vi "health_parameters.vi"(8 "error in\n(no error)":errorcluster, 10 "parameters":string[][](array[string]), 11 "hDin":T1={"nSignals"=0, "logname"="", "time"=timestamp(0 s since 1904-01-01), "dir"=path "", "adamSerial"={"port"="COM1", "timeout"=1000, "baud"=9600, "dataBits"=8, "stopBits"=10, "flowControl"=0, "parity"=0, "termChar"=FALSE, "checkSum"=FALSE}, "fiberSerial"={"port1"="COM1", "port2"="COM1", "timeout"=1000, "baud"=9600, "dataBits"=8, "stopBits"=10, "flowControl"=0, "parity"=0, "termChar"=FALSE, "checkSum"=FALSE, "fiber1On"=FALSE, "fiber2On"=FALSE}, "signal"={"src"=[], "id"=[], "ch"=[], "descrip"=[], "units"=[], "scale"=[], "hi"=[], "lo"=[], "rec"=[], "fault"=[], "val"=[]}, "teSerial"={"port"="COM1", "timeout"=1000, "baud"=9600, "dataBits"=8, "stopBits"=10, "flowControl"=0, "parity"=0, "termChar"=FALSE, "checkSum"=FALSE, "checkSumVal"=""}, "lograte"=0, "calSwitch"=FALSE, "logoffset"=0.0} {"teSerial"."stopBits" items=["1.0"=10, "1.5"=15, "2.0"=20]; "teSerial"."parity" items=["None", "Odd", "Even", "Mark", "Space"]; "teSerial"."flowControl" items=["None"=0, "XON/XOFF"=1, "RTS/CTS"=2, "DTR/DSR"=4]; "fiberSerial"."stopBits" items=["1.0"=10, "1.5"=15, "2.0"=20]; "fiberSerial"."parity" items=["None", "Odd", "Even", "Mark", "Space"]; "fiberSerial"."flowControl" items=["None"=0, "XON/XOFF"=1, "RTS/CTS"=2, "DTR/DSR"=4]; "adamSerial"."stopBits" items=["1.0"=10, "1.5"=15, "2.0"=20]; "adamSerial"."parity" items=["None", "Odd", "Even", "Mark", "Space"]; "adamSerial"."flowControl" items=["None"=0, "XON/XOFF"=1, "RTS/CTS"=2, "DTR/DSR"=4]}) -> (0 "error out":errorcluster, 3 "hDout":T1={"nSignals"=0, "logname"="", "time"=timestamp(0 s since 1904-01-01), "dir"=path "", "adamSerial"={"port"="COM1", "timeout"=1000, "baud"=9600, "dataBits"=8, "stopBits"=10, "flowControl"=0, "parity"=0, "termChar"=FALSE, "checkSum"=FALSE}, "fiberSerial"={"port1"="COM1", "port2"="COM1", "timeout"=1000, "baud"=9600, "dataBits"=8, "stopBits"=10, "flowControl"=0, "parity"=0, "termChar"=FALSE, "checkSum"=FALSE, "fiber1On"=FALSE, "fiber2On"=FALSE}, "signal"={"src"=[], "id"=[], "ch"=[], "descrip"=[], "units"=[], "scale"=[], "hi"=[], "lo"=[], "rec"=[], "fault"=[], "val"=[]}, "teSerial"={"port"="COM1", "timeout"=1000, "baud"=9600, "dataBits"=8, "stopBits"=10, "flowControl"=0, "parity"=0, "termChar"=FALSE, "checkSum"=FALSE, "checkSumVal"=""}, "lograte"=0, "calSwitch"=FALSE, "logoffset"=0.0} {"teSerial"."stopBits" items=["1.0"=10, "1.5"=15, "2.0"=20]; "teSerial"."parity" items=["None", "Odd", "Even", "Mark", "Space"]; "teSerial"."flowControl" items=["None"=0, "XON/XOFF"=1, "RTS/CTS"=2, "DTR/DSR"=4]; "fiberSerial"."stopBits" items=["1.0"=10, "1.5"=15, "2.0"=20]; "fiberSerial"."parity" items=["None", "Odd", "Even", "Mark", "Space"]; "fiberSerial"."flowControl" items=["None"=0, "XON/XOFF"=1, "RTS/CTS"=2, "DTR/DSR"=4]; "adamSerial"."stopBits" items=["1.0"=10, "1.5"=15, "2.0"=20]; "adamSerial"."parity" items=["None", "Odd", "Even", "Mark", "Space"]; "adamSerial"."flowControl" items=["None"=0, "XON/XOFF"=1, "RTS/CTS"=2, "DTR/DSR"=4]})   [LabVIEW 2018]
uses:
  health_Loop_Clust.ctl
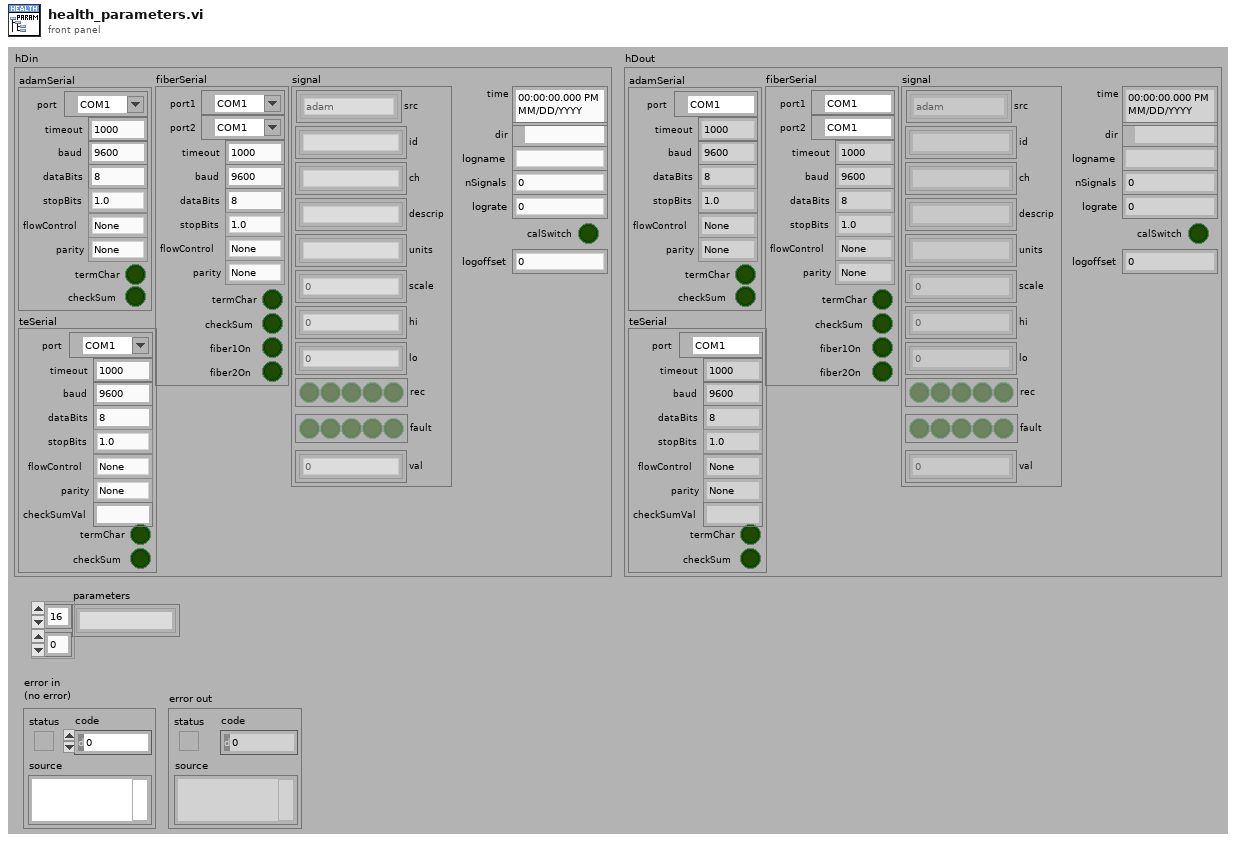
[diagram p1: front panel]
types:
  T1 = typedef "health_Loop_Clust.ctl" = cluster{"nSignals":i32, "logname":string, "time":timestamp, "dir":path, "adamSerial":cluster{"port":refnum<visa-resource-name>, "timeout":u32, "baud":u32, "dataBits":u16, "stopBits":u16, "flowControl":u16, "parity":u16, "termChar":bool, "checkSum":bool}, "fiberSerial":cluster{"port1":refnum<visa-resource-name>, "port2":refnum<visa-resource-name>, "timeout":u32, "baud":u32, "dataBits":u16, "stopBits":u16, "flowControl":u16, "parity":u16, "termChar":bool, "checkSum":bool, "fiber1On":bool, "fiber2On":bool}, "signal":cluster{"src":enum16{"adam", "fiber", "te"}[], "id":string[], "ch":string[], "descrip":string[], "units":string[], "scale":dbl[], "hi":dbl[], "lo":dbl[], "rec":bool[], "fault":bool[], "val":dbl[]}, "teSerial":cluster{"port":refnum<visa-resource-name>, "timeout":u32, "baud":u32, "dataBits":u16, "stopBits":u16, "flowControl":u16, "parity":u16, "termChar":bool, "checkSum":bool, "checkSumVal":string}, "lograte":u32, "calSwitch":bool, "logoffset":dbl}
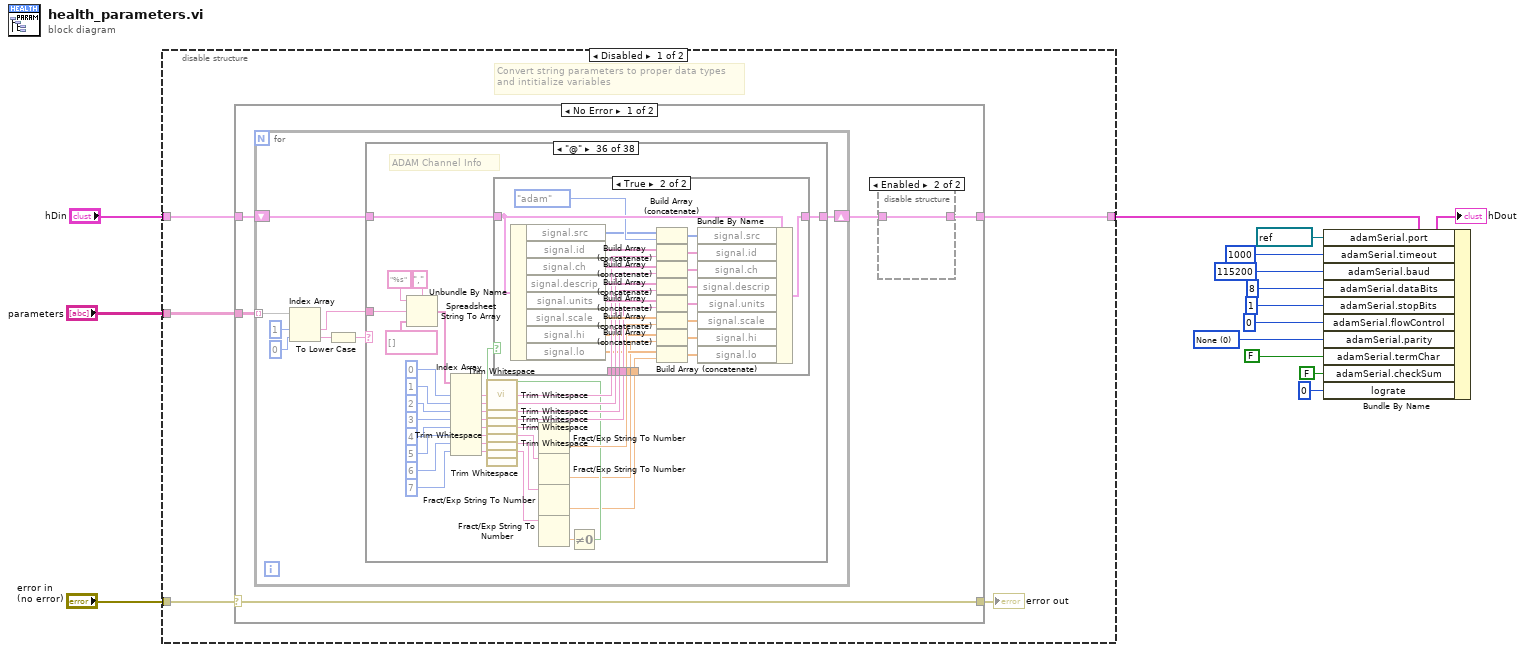
[diagram p0: block diagram]
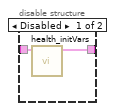
[diagram p2: hidden frame]
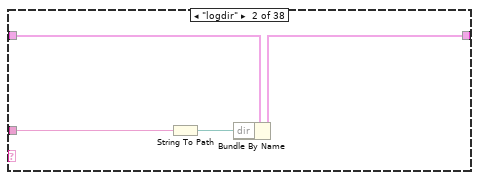
[diagram p4: hidden frame]
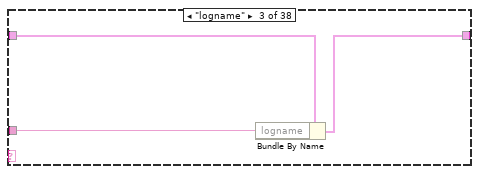
[diagram p5: hidden frame]
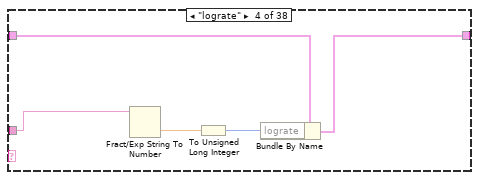
[diagram p6: hidden frame]
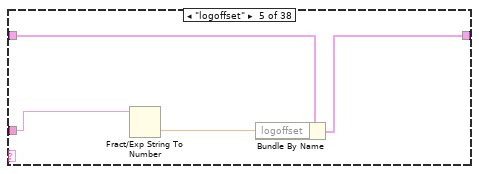
[diagram p7: hidden frame]
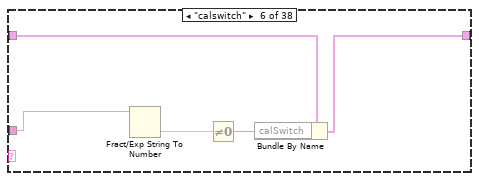
[diagram p8: hidden frame]
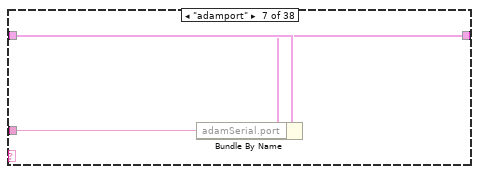
[diagram p9: hidden frame]
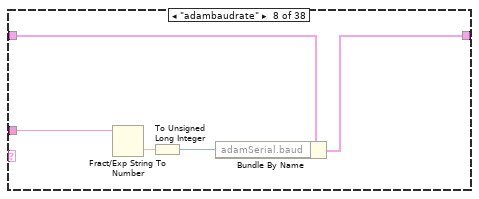
[diagram p10: hidden frame]
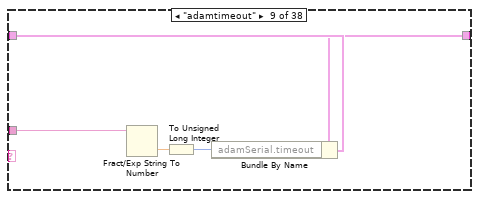
[diagram p11: hidden frame]
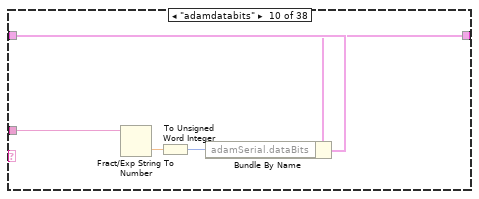
[diagram p12: hidden frame]
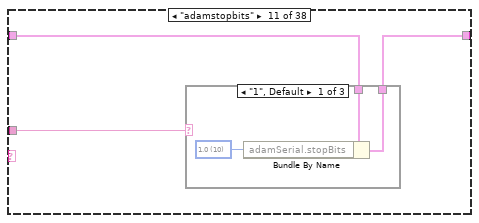
[diagram p13: hidden frame]
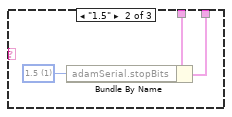
[diagram p14: hidden frame]
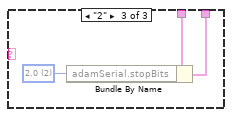
[diagram p15: hidden frame]
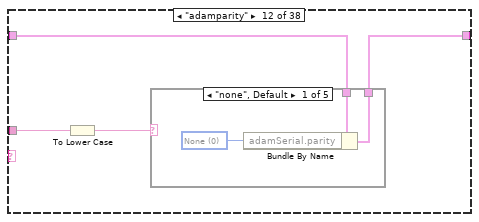
[diagram p16: hidden frame]
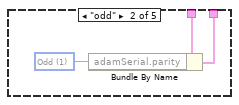
[diagram p17: hidden frame]
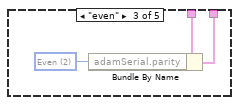
[diagram p18: hidden frame]
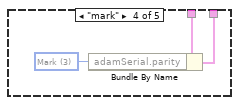
[diagram p19: hidden frame]
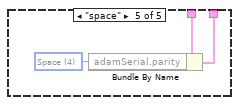
[diagram p20: hidden frame]
diagram:
  w1 = u16 0 items=["None", "Odd", "Even", "Mark", "Space"] ("parity")
  n1 = disable-structure shown="Disabled" {
    disable-tunnel: "error in\n(no error)" -> [w20 _]
    disable-tunnel: "parameters" -> [w18 _]
    disable-tunnel: "hDin" -> [w17 w487]
    disable-tunnel: [w16 w487] -> w12
    frame Disabled {
      # "Convert string parameters to proper data types\nand intitialize variables"
      n2 = case shown="No Error" w20 {
        selector: w20 -> [w25 w486]
        tunnel: [w25 w486] -> w19
        tunnel: [w21 w485] -> w16
        tunnel: w17 -> [w23 w485]
        tunnel: w18 -> [w24 _]
        frame No Error {
          n3 = for {
            shift-right: [w29] -> w22
            shift-left: w23 -> [w30]
            tunnel: w24 -> [w36] mode=indexing
            n4 = Index Array(array=w36, index #1=1 ("index"), index #2=0 ("index")) -> (element #1=w33:string, element #2=w32:string)
            n5 = To Lower Case(string=w32) -> (all lower case string=w31:string)
            n6 = case shown="\"@\"" w31 {
              tunnel: [w37 w40 w43 w48 w52 w57 w60 w65 w68 w73 w78 w91 w110 w128 w134 w137 w140 w145 w148 w153 w158 w171 w190 w208 w214 w217 w222 w225 w230 w235 w248 w267 w285 w291 w294 w319 w382 w445] -> w29
              tunnel: w33 -> [_ w39 w42 w47 w51 w56 w59 w66 w67 w75 w77 w90 w109 w127 w133 w136 w139 w146 w147 w155 w157 w170 w189 w207 w213 w216 w223 w224 w232 w234 w247 w266 w284 w290 w293 w328 w391 w454]
              tunnel: w30 -> [w37 w41 w44 w49 w53 w58 w61 w63 w69 w74 w79 w92 w111 w129 w135 w138 w141 w143 w149 w154 w159 w172 w191 w209 w215 w218 w220 w226 w231 w236 w249 w268 w286 w292 w295 w326 w389 w452]
              frame Default {
                # "Parameter Not Recognized"
              }
              frame "logdir" {
                n7 = String To Path(string=w39) -> (path=w38:path)
                n8 = Bundle By Name(cluster=w41, "dir"=w38) -> (w40:T1)
              }
              frame "logname" {
                n9 = Bundle By Name(cluster=w44, "logname"=w42) -> (w43:T1)
              }
              frame "lograte" {
                n10 = Fract/Exp String To Number(string=w47) -> (number=w45:dbl)  [unwired: 3 in, 1 out]
                n11 = To Unsigned Long Integer(number=w45) -> (unsigned 32bit integer=w46:u32)
                n12 = Bundle By Name(cluster=w49, "lograte"=w46) -> (w48:T1)
              }
              frame "logoffset" {
                n13 = Fract/Exp String To Number(string=w51) -> (number=w50:dbl)  [unwired: 3 in, 1 out]
                n14 = Bundle By Name(cluster=w53, "logoffset"=w50) -> (w52:T1)
              }
              frame "calswitch" {
                n15 = Fract/Exp String To Number(string=w56) -> (number=w54:dbl)  [unwired: 3 in, 1 out]
                n16 = Not Equal To 0?(x=w54) -> (x != 0?=w55:bool)
                n17 = Bundle By Name(cluster=w58, "calSwitch"=w55) -> (w57:T1)
              }
              frame "adamport" {
                n18 = Bundle By Name(cluster=w61, "adamSerial.port"=w59) -> (w60:T1)
              }
              frame "adambaudrate" {
                n19 = Fract/Exp String To Number(string=w66) -> (number=w64:dbl)  [unwired: 3 in, 1 out]
                n20 = To Unsigned Long Integer(number=w64) -> (unsigned 32bit integer=w62:u32)
                n21 = Bundle By Name(cluster=w63, "adamSerial.baud"=w62) -> (w65:T1)
              }
              frame "adamtimeout" {
                n22 = Fract/Exp String To Number(string=w67) -> (number=w70:dbl)  [unwired: 3 in, 1 out]
                n23 = To Unsigned Long Integer(number=w70) -> (unsigned 32bit integer=w71:u32)
                n24 = Bundle By Name(cluster=w69, "adamSerial.timeout"=w71) -> (w68:T1)
              }
              frame "adamdatabits" {
                n25 = Fract/Exp String To Number(string=w75) -> (number=w76:dbl)  [unwired: 3 in, 1 out]
                n26 = To Unsigned Word Integer(number=w76) -> (unsigned 16bit integer=w72:u16)
                n27 = Bundle By Name(cluster=w74, "adamSerial.dataBits"=w72) -> (w73:T1)
              }
              frame "adamstopbits" {
                n28 = case shown="\"1\", Default" w77 {
                  tunnel: w79 -> [w82 w85 w88]
                  tunnel: [w81 w84 w87] -> w78
                  frame "1", Default {
                    w80 = u16 10 items=["1.0"=10, "1.5"=15, "2.0"=20] ("stopBits")
                    n29 = Bundle By Name(cluster=w82, "adamSerial.stopBits"=w80) -> (w81:T1)
                  }
                  frame "1.5" {
                    w83 = u16 1 items=["1.0", "1.5", "2.0", "Other"] ("stopBits")
                    n30 = Bundle By Name(cluster=w85, "adamSerial.stopBits"=w83) -> (w84:T1)
                  }
                  frame "2" {
                    w86 = u16 2 items=["1.0", "1.5", "2.0", "Other"] ("stopBits")
                    n31 = Bundle By Name(cluster=w88, "adamSerial.stopBits"=w86) -> (w87:T1)
                  }
                }
              }
              frame "adamparity" {
                n32 = To Lower Case(string=w90) -> (all lower case string=w89:string)
                n33 = case shown="\"none\", Default" w89 {
                  tunnel: w92 -> [w95 w98 w101 w104 w107]
                  tunnel: [w94 w97 w100 w103 w106] -> w91
                  frame "none", Default {
                    w93 = u16 0 items=["None", "Odd", "Even", "Mark", "Space"] ("parity")
                    n34 = Bundle By Name(cluster=w95, "adamSerial.parity"=w93) -> (w94:T1)
                  }
                  frame "odd" {
                    w96 = u16 1 items=["None", "Odd", "Even", "Mark", "Space"] ("parity")
                    n35 = Bundle By Name(cluster=w98, "adamSerial.parity"=w96) -> (w97:T1)
                  }
                  frame "even" {
                    w99 = u16 2 items=["None", "Odd", "Even", "Mark", "Space"] ("parity")
                    n36 = Bundle By Name(cluster=w101, "adamSerial.parity"=w99) -> (w100:T1)
                  }
                  frame "mark" {
                    w102 = u16 3 items=["None", "Odd", "Even", "Mark", "Space"] ("parity")
                    n37 = Bundle By Name(cluster=w104, "adamSerial.parity"=w102) -> (w103:T1)
                  }
                  frame "space" {
                    w105 = u16 4 items=["None", "Odd", "Even", "Mark", "Space"] ("parity")
                    n38 = Bundle By Name(cluster=w107, "adamSerial.parity"=w105) -> (w106:T1)
                  }
                }
              }
              frame "adamflowcontrol" {
                n39 = To Lower Case(string=w109) -> (all lower case string=w108:string)
                n40 = case shown="\"none\", Default" w108 {
                  tunnel: w111 -> [w114 w117 w120 w123]
                  tunnel: [w113 w116 w119 w122] -> w110
                  frame "none", Default {
                    w112 = u16 0 items=["None"=0, "XON/XOFF"=1, "RTS/CTS"=2, "DTR/DSR"=4] ("flowControl")
                    n41 = Bundle By Name(cluster=w114, "adamSerial.flowControl"=w112) -> (w113:T1)
                  }
                  frame "xon/xoff" {
                    w115 = u16 1 items=["None"=0, "XON/XOFF"=1, "RTS/CTS"=2, "DTR/DSR"=4] ("flowControl")
                    n42 = Bundle By Name(cluster=w117, "adamSerial.flowControl"=w115) -> (w116:T1)
                  }
                  frame "rts/cts" {
                    w118 = u16 2 items=["None"=0, "XON/XOFF"=1, "RTS/CTS"=2, "DTR/DSR"=4] ("flowControl")
                    n43 = Bundle By Name(cluster=w120, "adamSerial.flowControl"=w118) -> (w119:T1)
                  }
                  frame "dtr/dsr" {
                    w121 = u16 4 items=["None"=0, "XON/XOFF"=1, "RTS/CTS"=2, "DTR/DSR"=4] ("flowControl")
                    n44 = Bundle By Name(cluster=w123, "adamSerial.flowControl"=w121) -> (w122:T1)
                  }
                }
              }
              frame "adamtermchar" {
                n45 = Fract/Exp String To Number(string=w127) -> (number=w126:dbl)  [unwired: 3 in, 1 out]
                n46 = Equal?(x=w126, y=1.0) -> (x = y?=w124:bool)
                n47 = Bundle By Name(cluster=w129, "adamSerial.termChar"=w124) -> (w128:T1)
              }
              frame "adamchecksum" {
                n48 = Fract/Exp String To Number(string=w133) -> (number=w132:dbl)  [unwired: 3 in, 1 out]
                n49 = Equal?(x=w132, y=1.0) -> (x = y?=w130:bool)
                n50 = Bundle By Name(cluster=w135, "adamSerial.checkSum"=w130) -> (w134:T1)
              }
              frame "fiberport1" {
                n51 = Bundle By Name(cluster=w138, "fiberSerial.port1"=w136) -> (w137:T1)
              }
              frame "fiberport2" {
                n52 = Bundle By Name(cluster=w141, "fiberSerial.port2"=w139) -> (w140:T1)
              }
              frame "fiberbaudrate" {
                n53 = Fract/Exp String To Number(string=w146) -> (number=w144:dbl)  [unwired: 3 in, 1 out]
                n54 = To Unsigned Long Integer(number=w144) -> (unsigned 32bit integer=w142:u32)
                n55 = Bundle By Name(cluster=w143, "fiberSerial.baud"=w142) -> (w145:T1)
              }
              frame "fibertimeout" {
                n56 = Fract/Exp String To Number(string=w147) -> (number=w150:dbl)  [unwired: 3 in, 1 out]
                n57 = To Unsigned Long Integer(number=w150) -> (unsigned 32bit integer=w151:u32)
                n58 = Bundle By Name(cluster=w149, "fiberSerial.timeout"=w151) -> (w148:T1)
              }
              frame "fiberdatabits" {
                n59 = Fract/Exp String To Number(string=w155) -> (number=w156:dbl)  [unwired: 3 in, 1 out]
                n60 = To Unsigned Word Integer(number=w156) -> (unsigned 16bit integer=w152:u16)
                n61 = Bundle By Name(cluster=w154, "fiberSerial.dataBits"=w152) -> (w153:T1)
              }
              frame "fiberstopbits" {
                n62 = case shown="\"1\", Default" w157 {
                  tunnel: w159 -> [w162 w165 w168]
                  tunnel: [w161 w164 w167] -> w158
                  frame "1", Default {
                    w160 = u16 10 items=["1.0"=10, "1.5"=15, "2.0"=20] ("stopBits")
                    n63 = Bundle By Name(cluster=w162, "fiberSerial.stopBits"=w160) -> (w161:T1)
                  }
                  frame "1.5" {
                    w163 = u16 1 items=["1.0", "1.5", "2.0", "Other"] ("stopBits")
                    n64 = Bundle By Name(cluster=w165, "fiberSerial.stopBits"=w163) -> (w164:T1)
                  }
                  frame "2" {
                    w166 = u16 2 items=["1.0", "1.5", "2.0", "Other"] ("stopBits")
                    n65 = Bundle By Name(cluster=w168, "fiberSerial.stopBits"=w166) -> (w167:T1)
                  }
                }
              }
              frame "fiberparity" {
                n66 = To Lower Case(string=w170) -> (all lower case string=w169:string)
                n67 = case shown="\"none\", Default" w169 {
                  tunnel: w172 -> [w175 w178 w181 w184 w187]
                  tunnel: [w174 w177 w180 w183 w186] -> w171
                  frame "none", Default {
                    w173 = u16 0 items=["None", "Odd", "Even", "Mark", "Space"] ("parity")
                    n68 = Bundle By Name(cluster=w175, "fiberSerial.parity"=w173) -> (w174:T1)
                  }
                  frame "odd" {
                    w176 = u16 1 items=["None", "Odd", "Even", "Mark", "Space"] ("parity")
                    n69 = Bundle By Name(cluster=w178, "fiberSerial.parity"=w176) -> (w177:T1)
                  }
                  frame "even" {
                    w179 = u16 2 items=["None", "Odd", "Even", "Mark", "Space"] ("parity")
                    n70 = Bundle By Name(cluster=w181, "fiberSerial.parity"=w179) -> (w180:T1)
                  }
                  frame "mark" {
                    w182 = u16 3 items=["None", "Odd", "Even", "Mark", "Space"] ("parity")
                    n71 = Bundle By Name(cluster=w184, "fiberSerial.parity"=w182) -> (w183:T1)
                  }
                  frame "space" {
                    w185 = u16 4 items=["None", "Odd", "Even", "Mark", "Space"] ("parity")
                    n72 = Bundle By Name(cluster=w187, "fiberSerial.parity"=w185) -> (w186:T1)
                  }
                }
              }
              frame "fiberflowcontrol" {
                n73 = To Lower Case(string=w189) -> (all lower case string=w188:string)
                n74 = case shown="\"none\", Default" w188 {
                  tunnel: w191 -> [w194 w197 w200 w203]
                  tunnel: [w193 w196 w199 w202] -> w190
                  frame "none", Default {
                    w192 = u16 0 items=["None"=0, "XON/XOFF"=1, "RTS/CTS"=2, "DTR/DSR"=4] ("flowControl")
                    n75 = Bundle By Name(cluster=w194, "fiberSerial.flowControl"=w192) -> (w193:T1)
                  }
                  frame "xon/xoff" {
                    w195 = u16 1 items=["None"=0, "XON/XOFF"=1, "RTS/CTS"=2, "DTR/DSR"=4] ("flowControl")
                    n76 = Bundle By Name(cluster=w197, "fiberSerial.flowControl"=w195) -> (w196:T1)
                  }
                  frame "rts/cts" {
                    w198 = u16 2 items=["None"=0, "XON/XOFF"=1, "RTS/CTS"=2, "DTR/DSR"=4] ("flowControl")
                    n77 = Bundle By Name(cluster=w200, "fiberSerial.flowControl"=w198) -> (w199:T1)
                  }
                  frame "dtr/dsr" {
                    w201 = u16 4 items=["None"=0, "XON/XOFF"=1, "RTS/CTS"=2, "DTR/DSR"=4] ("flowControl")
                    n78 = Bundle By Name(cluster=w203, "fiberSerial.flowControl"=w201) -> (w202:T1)
                  }
                }
              }
              frame "fibertermchar" {
                n79 = Fract/Exp String To Number(string=w207) -> (number=w206:dbl)  [unwired: 3 in, 1 out]
                n80 = Equal?(x=w206, y=1.0) -> (x = y?=w204:bool)
                n81 = Bundle By Name(cluster=w209, "fiberSerial.termChar"=w204) -> (w208:T1)
              }
              frame "fiberchecksum" {
                n82 = Fract/Exp String To Number(string=w213) -> (number=w212:dbl)  [unwired: 3 in, 1 out]
                n83 = Equal?(x=w212, y=1.0) -> (x = y?=w210:bool)
                n84 = Bundle By Name(cluster=w215, "fiberSerial.checkSum"=w210) -> (w214:T1)
              }
              frame "teport1" {
                n85 = Bundle By Name(cluster=w218, "teSerial.port"=w216) -> (w217:T1)
              }
              frame "tebaudrate" {
                n86 = Fract/Exp String To Number(string=w223) -> (number=w221:dbl)  [unwired: 3 in, 1 out]
                n87 = To Unsigned Long Integer(number=w221) -> (unsigned 32bit integer=w219:u32)
                n88 = Bundle By Name(cluster=w220, "teSerial.baud"=w219) -> (w222:T1)
              }
              frame "tetimeout" {
                n89 = Fract/Exp String To Number(string=w224) -> (number=w227:dbl)  [unwired: 3 in, 1 out]
                n90 = To Unsigned Long Integer(number=w227) -> (unsigned 32bit integer=w228:u32)
                n91 = Bundle By Name(cluster=w226, "teSerial.timeout"=w228) -> (w225:T1)
              }
              frame "tedatabits" {
                n92 = Fract/Exp String To Number(string=w232) -> (number=w233:dbl)  [unwired: 3 in, 1 out]
                n93 = To Unsigned Word Integer(number=w233) -> (unsigned 16bit integer=w229:u16)
                n94 = Bundle By Name(cluster=w231, "teSerial.dataBits"=w229) -> (w230:T1)
              }
              frame "testopbits" {
                n95 = case shown="\"2\"" w234 {
                  tunnel: w236 -> [w239 w242 w245]
                  tunnel: [w238 w241 w244] -> w235
                  frame "1", Default {
                    w237 = u16 10 items=["1.0"=10, "1.5"=15, "2.0"=20] ("stopBits")
                    n96 = Bundle By Name(cluster=w239, "teSerial.stopBits"=w237) -> (w238:T1)
                  }
                  frame "1.5" {
                    w240 = u16 1 items=["1.0", "1.5", "2.0", "Other"] ("stopBits")
                    n97 = Bundle By Name(cluster=w242, "teSerial.stopBits"=w240) -> (w241:T1)
                  }
                  frame "2" {
                    w243 = u16 2 items=["1.0", "1.5", "2.0", "Other"] ("stopBits")
                    n98 = Bundle By Name(cluster=w245, "teSerial.stopBits"=w243) -> (w244:T1)
                  }
                }
              }
              frame "teparity" {
                n99 = To Lower Case(string=w247) -> (all lower case string=w246:string)
                n100 = case shown="\"none\", Default" w246 {
                  tunnel: w249 -> [w252 w255 w258 w261 w264]
                  tunnel: [w251 w254 w257 w260 w263] -> w248
                  frame "none", Default {
                    w250 = u16 0 items=["None", "Odd", "Even", "Mark", "Space"] ("parity")
                    n101 = Bundle By Name(cluster=w252, "teSerial.parity"=w250) -> (w251:T1)
                  }
                  frame "odd" {
                    w253 = u16 1 items=["None", "Odd", "Even", "Mark", "Space"] ("parity")
                    n102 = Bundle By Name(cluster=w255, "teSerial.parity"=w253) -> (w254:T1)
                  }
                  frame "even" {
                    w256 = u16 2 items=["None", "Odd", "Even", "Mark", "Space"] ("parity")
                    n103 = Bundle By Name(cluster=w258, "teSerial.parity"=w256) -> (w257:T1)
                  }
                  frame "mark" {
                    w259 = u16 3 items=["None", "Odd", "Even", "Mark", "Space"] ("parity")
                    n104 = Bundle By Name(cluster=w261, "teSerial.parity"=w259) -> (w260:T1)
                  }
                  frame "space" {
                    w262 = u16 4 items=["None", "Odd", "Even", "Mark", "Space"] ("parity")
                    n105 = Bundle By Name(cluster=w264, "teSerial.parity"=w262) -> (w263:T1)
                  }
                }
              }
              frame "teflowcontrol" {
                n106 = To Lower Case(string=w266) -> (all lower case string=w265:string)
                n107 = case shown="\"dtr/dsr\"" w265 {
                  tunnel: w268 -> [w271 w274 w277 w280]
                  tunnel: [w270 w273 w276 w279] -> w267
                  frame "none", Default {
                    w269 = u16 0 items=["None"=0, "XON/XOFF"=1, "RTS/CTS"=2, "DTR/DSR"=4] ("flowControl")
                    n108 = Bundle By Name(cluster=w271, "teSerial.flowControl"=w269) -> (w270:T1)
                  }
                  frame "xon/xoff" {
                    w272 = u16 1 items=["None"=0, "XON/XOFF"=1, "RTS/CTS"=2, "DTR/DSR"=4] ("flowControl")
                    n109 = Bundle By Name(cluster=w274, "teSerial.flowControl"=w272) -> (w273:T1)
                  }
                  frame "rts/cts" {
                    w275 = u16 2 items=["None"=0, "XON/XOFF"=1, "RTS/CTS"=2, "DTR/DSR"=4] ("flowControl")
                    n110 = Bundle By Name(cluster=w277, "teSerial.flowControl"=w275) -> (w276:T1)
                  }
                  frame "dtr/dsr" {
                    w278 = u16 4 items=["None"=0, "XON/XOFF"=1, "RTS/CTS"=2, "DTR/DSR"=4] ("flowControl")
                    n111 = Bundle By Name(cluster=w280, "teSerial.flowControl"=w278) -> (w279:T1)
                  }
                }
              }
              frame "tetermchar" {
                n112 = Fract/Exp String To Number(string=w284) -> (number=w283:dbl)  [unwired: 3 in, 1 out]
                n113 = Equal?(x=w283, y=1.0) -> (x = y?=w281:bool)
                n114 = Bundle By Name(cluster=w286, "teSerial.termChar"=w281) -> (w285:T1)
              }
              frame "techecksum" {
                n115 = Fract/Exp String To Number(string=w290) -> (number=w289:dbl)  [unwired: 3 in, 1 out]
                n116 = Equal?(x=w289, y=1.0) -> (x = y?=w287:bool)
                n117 = Bundle By Name(cluster=w292, "teSerial.checkSum"=w287) -> (w291:T1)
              }
              frame "techecksumval" {
                n118 = Bundle By Name(cluster=w295, "teSerial.checkSumVal"=w293) -> (w294:T1)
              }
              frame "@" {
                # "ADAM Channel Info"
                n119 = Spreadsheet String To Array(delimiter (Tab)=",", format string="%s", spreadsheet string=w328, array type (2D Dbl)=string[] []) -> (array=w306:string[])
                n120 = Index Array(array=w306, index #1=0 ("index"), index #2=1 ("index"), index #3=2 ("index"), index #4=3 ("index"), index #5=4 ("index"), index #6=5 ("index"), index #7=6 ("index"), index #8=7 ("index")) -> (element #1=w318:string, element #2=w316:string, element #3=w314:string, element #4=w312:string, element #5=w311:string, element #6=w310:string, element #7=w302:string, element #8=w301:string)
                n121 = call <vilib>:"Trim Whitespace.vi"("string"=w318) -> ("trimmed string"=w317:string)  [unwired: 1 in]
                n122 = call <vilib>:"Trim Whitespace.vi"("string"=w316) -> ("trimmed string"=w315:string)  [unwired: 1 in]
                n123 = call <vilib>:"Trim Whitespace.vi"("string"=w314) -> ("trimmed string"=w313:string)  [unwired: 1 in]
                n124 = call <vilib>:"Trim Whitespace.vi"("string"=w312) -> ("trimmed string"=w309:string)  [unwired: 1 in]
                n125 = call <vilib>:"Trim Whitespace.vi"("string"=w311) -> ("trimmed string"=w308:string)  [unwired: 1 in]
                n126 = call <vilib>:"Trim Whitespace.vi"("string"=w310) -> ("trimmed string"=w300:string)  [unwired: 1 in]
                n127 = call <vilib>:"Trim Whitespace.vi"("string"=w302) -> ("trimmed string"=w299:string)  [unwired: 1 in]
                n128 = call <vilib>:"Trim Whitespace.vi"("string"=w301) -> ("trimmed string"=w298:string)  [unwired: 1 in]
                n129 = Fract/Exp String To Number(string=w308) -> (number=w325:dbl)  [unwired: 3 in, 1 out]
                n130 = Fract/Exp String To Number(string=w300) -> (number=w304:dbl)  [unwired: 3 in, 1 out]
                n131 = Fract/Exp String To Number(string=w299) -> (number=w303:dbl)  [unwired: 3 in, 1 out]
                n132 = Fract/Exp String To Number(string=w298) -> (number=w307:dbl)  [unwired: 3 in, 1 out]
                n133 = Not Equal To 0?(x=w307) -> (x != 0?=w305:bool)
                n134 = case shown="True" w305 {
                  tunnel: w326 -> [w332 w358]
                  tunnel: w325 -> [_ w342]
                  tunnel: [w332 w347] -> w319
                  tunnel: w317 -> [_ w346]
                  tunnel: w315 -> [_ w345]
                  tunnel: w313 -> [_ w344]
                  tunnel: w309 -> [_ w343]
                  tunnel: w304 -> [_ w337]
                  tunnel: w303 -> [_ w336]
                  frame False {
                    # "Do not append"
                  }
                  frame True {
                    n135 = Unbundle By Name(w358) -> ("signal.src"=w333:enum16{"adam", "fiber", "te"}[], "signal.id"=w357:string[], "signal.ch"=w355:string[], "signal.descrip"=w353:string[], "signal.units"=w352:string[], "signal.scale"=w351:dbl[], "signal.hi"=w341:dbl[], "signal.lo"=w340:dbl[])
                    n136 = Build Array (concatenate)(w333, enum16{"adam", "fiber"}."adam" ("src")) -> (w334:enum16{"adam", "fiber", "te"}[])
                    n137 = Build Array (concatenate)(w357, w346) -> (w356:string[])
                    n138 = Build Array (concatenate)(w355, w345) -> (w354:string[])
                    n139 = Build Array (concatenate)(w353, w344) -> (w348:string[])
                    n140 = Build Array (concatenate)(w352, w343) -> (w349:string[])
                    n141 = Build Array (concatenate)(w351, w342) -> (w350:dbl[])
                    n142 = Build Array (concatenate)(w341, w337) -> (w339:dbl[])
                    n143 = Build Array (concatenate)(w340, w336) -> (w338:dbl[])
                    n144 = Bundle By Name(cluster=w358, "signal.src"=w334, "signal.id"=w356, "signal.ch"=w354, "signal.descrip"=w348, "signal.units"=w349, "signal.scale"=w350, "signal.hi"=w339, "signal.lo"=w338) -> (w347:T1)
                  }
                }
              }
              frame "%" {
                # "Fiber Channel Info"
                n145 = Spreadsheet String To Array(delimiter (Tab)=",", format string="%s", spreadsheet string=w391, array type (2D Dbl)=string[] []) -> (array=w369:string[])
                n146 = Index Array(array=w369, index #1=0 ("index"), index #2=1 ("index"), index #3=2 ("index"), index #4=3 ("index"), index #5=4 ("index"), index #6=5 ("index"), index #7=6 ("index"), index #8=7 ("index")) -> (element #1=w381:string, element #2=w379:string, element #3=w377:string, element #4=w375:string, element #5=w374:string, element #6=w373:string, element #7=w365:string, element #8=w364:string)
                n147 = call <vilib>:"Trim Whitespace.vi"("string"=w381) -> ("trimmed string"=w380:string)  [unwired: 1 in]
                n148 = call <vilib>:"Trim Whitespace.vi"("string"=w379) -> ("trimmed string"=w378:string)  [unwired: 1 in]
                n149 = call <vilib>:"Trim Whitespace.vi"("string"=w377) -> ("trimmed string"=w376:string)  [unwired: 1 in]
                n150 = call <vilib>:"Trim Whitespace.vi"("string"=w375) -> ("trimmed string"=w372:string)  [unwired: 1 in]
                n151 = call <vilib>:"Trim Whitespace.vi"("string"=w374) -> ("trimmed string"=w371:string)  [unwired: 1 in]
                n152 = call <vilib>:"Trim Whitespace.vi"("string"=w373) -> ("trimmed string"=w363:string)  [unwired: 1 in]
                n153 = call <vilib>:"Trim Whitespace.vi"("string"=w365) -> ("trimmed string"=w362:string)  [unwired: 1 in]
                n154 = call <vilib>:"Trim Whitespace.vi"("string"=w364) -> ("trimmed string"=w361:string)  [unwired: 1 in]
                n155 = Fract/Exp String To Number(string=w371) -> (number=w388:dbl)  [unwired: 3 in, 1 out]
                n156 = Fract/Exp String To Number(string=w363) -> (number=w367:dbl)  [unwired: 3 in, 1 out]
                n157 = Fract/Exp String To Number(string=w362) -> (number=w366:dbl)  [unwired: 3 in, 1 out]
                n158 = Fract/Exp String To Number(string=w361) -> (number=w370:dbl)  [unwired: 3 in, 1 out]
                n159 = Not Equal To 0?(x=w370) -> (x != 0?=w368:bool)
                n160 = case shown="True" w368 {
                  tunnel: w389 -> [w395 w421]
                  tunnel: w388 -> [_ w405]
                  tunnel: [w395 w410] -> w382
                  tunnel: w380 -> [_ w409]
                  tunnel: w378 -> [_ w408]
                  tunnel: w376 -> [_ w407]
                  tunnel: w372 -> [_ w406]
                  tunnel: w367 -> [_ w400]
                  tunnel: w366 -> [_ w399]
                  frame False {
                    # "Do not append"
                  }
                  frame True {
                    n161 = Unbundle By Name(w421) -> ("signal.src"=w396:enum16{"adam", "fiber", "te"}[], "signal.id"=w420:string[], "signal.ch"=w418:string[], "signal.descrip"=w416:string[], "signal.units"=w415:string[], "signal.scale"=w414:dbl[], "signal.hi"=w404:dbl[], "signal.lo"=w403:dbl[])
                    n162 = Build Array (concatenate)(w396, enum16{"adam", "fiber"}."fiber" ("src")) -> (w397:enum16{"adam", "fiber", "te"}[])
                    n163 = Build Array (concatenate)(w420, w409) -> (w419:string[])
                    n164 = Build Array (concatenate)(w418, w408) -> (w417:string[])
                    n165 = Build Array (concatenate)(w416, w407) -> (w411:string[])
                    n166 = Build Array (concatenate)(w415, w406) -> (w412:string[])
                    n167 = Build Array (concatenate)(w414, w405) -> (w413:dbl[])
                    n168 = Build Array (concatenate)(w404, w400) -> (w402:dbl[])
                    n169 = Build Array (concatenate)(w403, w399) -> (w401:dbl[])
                    n170 = Bundle By Name(cluster=w421, "signal.src"=w397, "signal.id"=w419, "signal.ch"=w417, "signal.descrip"=w411, "signal.units"=w412, "signal.scale"=w413, "signal.hi"=w402, "signal.lo"=w401) -> (w410:T1)
                  }
                }
              }
              frame "&" {
                # "TE Channel Info"
                n171 = Spreadsheet String To Array(delimiter (Tab)=",", format string="%s", spreadsheet string=w454, array type (2D Dbl)=string[] []) -> (array=w432:string[])
                n172 = Index Array(array=w432, index #1=0 ("index"), index #2=1 ("index"), index #3=2 ("index"), index #4=3 ("index"), index #5=4 ("index"), index #6=5 ("index"), index #7=6 ("index"), index #8=7 ("index")) -> (element #1=w444:string, element #2=w442:string, element #3=w440:string, element #4=w438:string, element #5=w437:string, element #6=w436:string, element #7=w428:string, element #8=w427:string)
                n173 = call <vilib>:"Trim Whitespace.vi"("string"=w444) -> ("trimmed string"=w443:string)  [unwired: 1 in]
                n174 = call <vilib>:"Trim Whitespace.vi"("string"=w442) -> ("trimmed string"=w441:string)  [unwired: 1 in]
                n175 = call <vilib>:"Trim Whitespace.vi"("string"=w440) -> ("trimmed string"=w439:string)  [unwired: 1 in]
                n176 = call <vilib>:"Trim Whitespace.vi"("string"=w438) -> ("trimmed string"=w435:string)  [unwired: 1 in]
                n177 = call <vilib>:"Trim Whitespace.vi"("string"=w437) -> ("trimmed string"=w434:string)  [unwired: 1 in]
                n178 = call <vilib>:"Trim Whitespace.vi"("string"=w436) -> ("trimmed string"=w426:string)  [unwired: 1 in]
                n179 = call <vilib>:"Trim Whitespace.vi"("string"=w428) -> ("trimmed string"=w425:string)  [unwired: 1 in]
                n180 = call <vilib>:"Trim Whitespace.vi"("string"=w427) -> ("trimmed string"=w424:string)  [unwired: 1 in]
                n181 = Fract/Exp String To Number(string=w434) -> (number=w451:dbl)  [unwired: 3 in, 1 out]
                n182 = Fract/Exp String To Number(string=w426) -> (number=w430:dbl)  [unwired: 3 in, 1 out]
                n183 = Fract/Exp String To Number(string=w425) -> (number=w429:dbl)  [unwired: 3 in, 1 out]
                n184 = Fract/Exp String To Number(string=w424) -> (number=w433:dbl)  [unwired: 3 in, 1 out]
                n185 = Not Equal To 0?(x=w433) -> (x != 0?=w431:bool)
                n186 = case shown="True" w431 {
                  tunnel: w452 -> [w458 w484]
                  tunnel: w451 -> [_ w468]
                  tunnel: [w458 w473] -> w445
                  tunnel: w443 -> [_ w472]
                  tunnel: w441 -> [_ w471]
                  tunnel: w439 -> [_ w470]
                  tunnel: w435 -> [_ w469]
                  tunnel: w430 -> [_ w463]
                  tunnel: w429 -> [_ w462]
                  frame False {
                    # "Do not append"
                  }
                  frame True {
                    n187 = Unbundle By Name(w484) -> ("signal.src"=w459:enum16{"adam", "fiber", "te"}[], "signal.id"=w483:string[], "signal.ch"=w481:string[], "signal.descrip"=w479:string[], "signal.units"=w478:string[], "signal.scale"=w477:dbl[], "signal.hi"=w467:dbl[], "signal.lo"=w466:dbl[])
                    n188 = Build Array (concatenate)(w459, enum16{"adam", "fiber", "te"}."te" ("src")) -> (w460:enum16{"adam", "fiber", "te"}[])
                    n189 = Build Array (concatenate)(w483, w472) -> (w482:string[])
                    n190 = Build Array (concatenate)(w481, w471) -> (w480:string[])
                    n191 = Build Array (concatenate)(w479, w470) -> (w474:string[])
                    n192 = Build Array (concatenate)(w478, w469) -> (w475:string[])
                    n193 = Build Array (concatenate)(w477, w468) -> (w476:dbl[])
                    n194 = Build Array (concatenate)(w467, w463) -> (w465:dbl[])
                    n195 = Build Array (concatenate)(w466, w462) -> (w464:dbl[])
                    n196 = Bundle By Name(cluster=w484, "signal.src"=w460, "signal.id"=w482, "signal.ch"=w480, "signal.descrip"=w474, "signal.units"=w475, "signal.scale"=w476, "signal.hi"=w465, "signal.lo"=w464) -> (w473:T1)
                  }
                }
              }
            }
          }
          n197 = disable-structure shown="Enabled" {
            disable-tunnel: w22 -> [w27 w28]
            disable-tunnel: [w26 w28] -> w21
            frame Disabled {
              n198 = call "health_initVars.vi"("hDin"=w27) -> ("hDout"=w26:T1)  [unwired: 10 in]
            }
            frame Enabled {
            }
          }
        }
        frame Error {
        }
      }
      "error out" <- w19
    }
    frame Enabled {
      # "Not reading from file anymore. Explicitly setting ADAM config here--------------------------->\nLuke 1-22-2019"
    }
  }
  n199 = Bundle By Name(cluster=w12, "adamSerial.port"=refnum<visa-resource-name> "Port1", "adamSerial.timeout"=u32 1000, "adamSerial.baud"=u32 115200, "adamSerial.dataBits"=u16 8, "adamSerial.stopBits"=u16 1, "adamSerial.flowControl"=u16 0, "adamSerial.parity"=w1, "adamSerial.termChar"=FALSE, "adamSerial.checkSum"=FALSE, "lograte"=u32 0) -> (→"hDout":T1)
